vi "Set AI filter.vi"(8 "error in (no error)":errorcluster, 11 "Enable All Low Pass Filter":bool) -> (0 "error out":errorcluster)   [LabVIEW 2024]
uses:
  <vilib>/rvi/eio/common/nirviEmuTemplatePropertySet_errors.vi
  <vilib>/eio/EIOPropertyNode/EIOPropertyNode.xnode
  <vilib>/rvi/eio/common/nirviEmuTemplatePropertyGet_errors.vi
  <vilib>/rvi/eio/common/nirviEmuTemplatePropertyGet_noerrors.vi
  <vilib>/rvi/eio/common/nirviEmuTemplatePropertySet_noerrors.vi
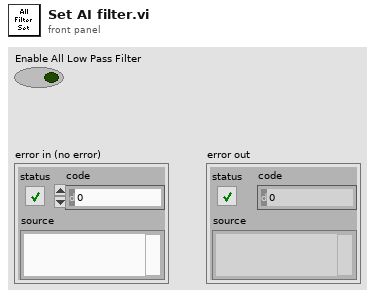
[diagram p1: front panel]
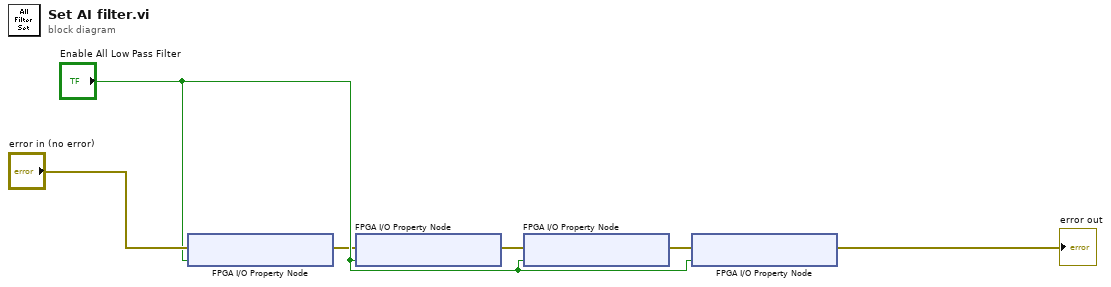
[diagram p0: block diagram]
diagram:
  n1 = xnode "FPGA I/O Property Node"("error in"="error in (no error)", "Enable Analog Filter"="Enable All Low Pass Filter") -> ("error out"=w1:errorcluster)  [unwired: 1 in, 1 out]
  n2 = xnode "FPGA I/O Property Node"("error in"=w1, "Enable Analog Filter"="Enable All Low Pass Filter") -> ("error out"=w2:errorcluster)  [unwired: 1 in, 1 out]
  n3 = xnode "FPGA I/O Property Node"("error in"=w2, "Enable Analog Filter"="Enable All Low Pass Filter") -> ("error out"=w3:errorcluster)  [unwired: 1 in, 1 out]
  n4 = xnode "FPGA I/O Property Node"("error in"=w3, "Enable Analog Filter"="Enable All Low Pass Filter") -> ("error out"=→"error out":errorcluster)  [unwired: 1 in, 1 out]
